vi "Add Elements to Meas Plugin UI.vi"(11 "error in (no error)":errorcluster) -> (15 "error out":errorcluster)   [LabVIEW 2021, in "Converter.lvlib"]
uses:
  Converter.lvlib
  Converter Reusables/Converter Reusables.lvlib
  Path Functions/Path Functions.lvlib
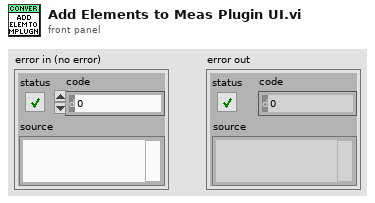
[diagram p1: front panel]
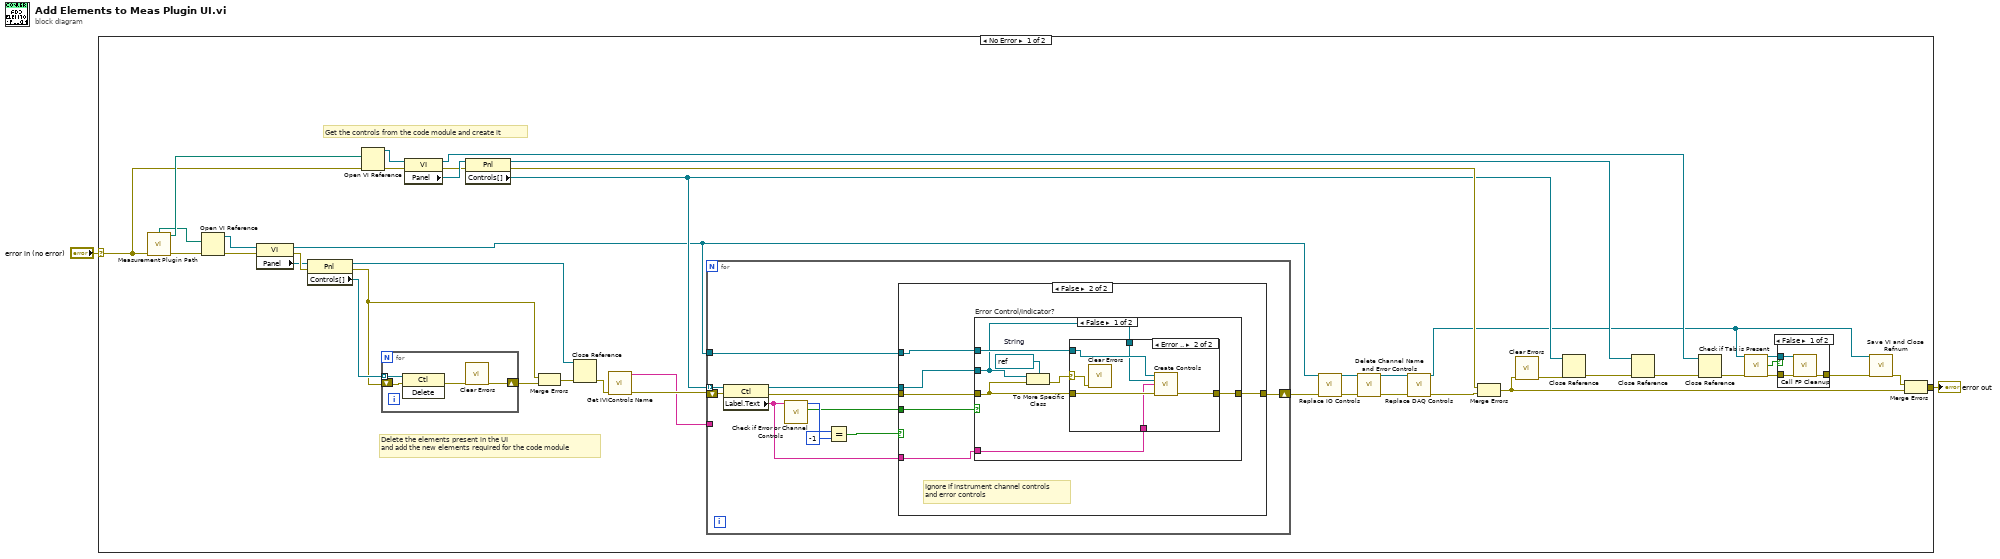
[diagram p0: block diagram]
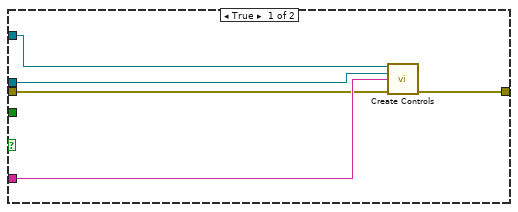
[diagram p2: hidden frame]
diagram:
  n1 = case shown="No Error" "error in (no error)" {
    selector: "error in (no error)" -> [w4 w91]
    tunnel: [w36 w91] -> w2
    frame No Error {
      # "Get the controls from the code module and create it"
      # "Delete the elements present in the UI\nand add the new elements required for the code module"
      n2 = call "Measurement Plugin Path.vi"("error in (no error)"=w4) -> ("Measurement UI"=w5:path, "New Code Module"=w6:path, "error out"=w3:errorcluster)  [unwired: 2 in, 10 out]
      n3 = Open VI Reference(vi path=w5, error in (no error)=w3) -> (vi reference=w24:refnum<vi>, error out=w45:errorcluster)  [unwired: 4 in]
      n4 = property class="VI"(reference=w24, error in=w45) -> (reference out=w28:refnum<vi>, error out=w44:errorcluster, "Panel"=w30:refnum<vi>)
      n5 = property class="Pnl"(reference=w30, error in=w44) -> (reference out=w29:refnum<vi>, error out=w15:errorcluster, "Controls[]"=w43:refnum<vi>[])
      n6 = Open VI Reference(vi path=w6, error in (no error)=w4) -> (vi reference=w21:refnum<vi>, error out=w38:errorcluster)  [unwired: 4 in]
      n7 = for {
        tunnel: w43 -> [w49] mode=indexing
        shift-right: [w46] -> w42
        shift-left: w15 -> [w48]
        n8 = invoke class="Ctl" method="Delete"(reference=w49, error in=w48) -> (error out=w47:errorcluster)  [unwired: 1 in, 2 out]
        n9 = call <vilib>:"Clear Errors.vi"("error in (no error)"=w47) -> ("error out"=w46:errorcluster)  [unwired: 5 in, 1 out]
      }
      n10 = property class="VI"(reference=w21, error in=w38) -> (reference out=w20:refnum<vi>, error out=w37:errorcluster, "Panel"=w39:refnum<vi>)
      n11 = property class="Pnl"(reference=w39, error in=w37) -> (reference out=w19:refnum<vi>, error out=w41:errorcluster, "Controls[]"=w40:refnum<vi>[])
      n12 = Merge Errors(w15, w42) -> (w16:errorcluster)
      n13 = Close Reference(reference=w29, error in (no error)=w16) -> (error out=w23:errorcluster)
      n14 = call "Get IVIControls Name.vi"("error in (no error)"=w23) -> ("Control Names Out"=w31:string[], "error out"=w32:errorcluster)  [unwired: 12 in, 1 out]
      n15 = for {
        tunnel: w28 -> [w60]
        tunnel: w40 -> [w58] mode=indexing
        shift-right: [w59] -> w27
        shift-left: w32 -> [w57]
        tunnel: w31 -> [_]
        n16 = property class="Ctl"(reference=w58, error in=w57) -> (reference out=w55:refnum<vi>, error out=w54:errorcluster, "Label.Text"=w56:string)
        n17 = call "Check if Error or Channel Controls.vi"("Label.Text"=w56) -> ("Error?"=w50:bool, "offset past match"=w53:i32)  [unwired: 9 in]
        n18 = Equal?(x=w53, y=-1) -> (x = y?=w51:bool)
        n19 = case shown="False" w51 {
          tunnel: w60 -> [w65 w68]
          tunnel: [w64 w66] -> w59
          tunnel: w55 -> [w62 w71]
          tunnel: w54 -> [w61 w70]
          tunnel: w56 -> [w63 w67]
          tunnel: w50 -> [_ w69]
          frame True {
            n20 = call "Create Controls.vi"("VI in"=w65, "Ctl Refnum"=w62, "Control Label"=w63, "error in (no error)"=w61) -> ("error out"=w64:errorcluster)  [unwired: 11 in]
          }
          frame False {
            # "Ignore if instrument channel controls\nand error controls"
            n21 = case "Error Control/Indicator?" shown="False" w69 {
              tunnel: w71 -> [w74 _]
              tunnel: w70 -> [w77 w86]
              tunnel: w68 -> [w75 _]
              tunnel: w67 -> [w73 _]
              tunnel: [w72 w86] -> w66
              frame False {
                w78 = refnum<vi> refnum  # String
                n22 = To More Specific Class(target class=w78, reference=w74, error in=w77) -> (error out=w76:errorcluster)  [unwired: 1 out]
                n23 = case shown="Error .." w76 {
                  selector: w76 -> [_ w80]
                  tunnel: w77 -> [w79 w85]
                  tunnel: w75 -> [_ w84]
                  tunnel: w74 -> [_ w83]
                  tunnel: w73 -> [_ w82]
                  tunnel: [w79 w81] -> w72
                  frame No Error {
                  }
                  frame Error {
                    n24 = call <vilib>:"Clear Errors.vi"("error in (no error)"=w80) -> ()  [unwired: 5 in, 2 out]
                    n25 = call "Create Controls.vi"("VI in"=w84, "Ctl Refnum"=w83, "Control Label"=w82, "error in (no error)"=w85) -> ("error out"=w81:errorcluster)  [unwired: 11 in]
                  }
                }
              }
              frame True {
              }
            }
          }
        }
      }
      n26 = call "Replace IO Controls.vi"("VI in"=w28, "error in (no error)"=w27) -> ("VI out"=w26:refnum<vi>, "error out"=w25:errorcluster)  [unwired: 12 in]
      n27 = call "Delete Channel Name and Error Controls.vi"("VI in"=w26, "error in (no error)"=w25) -> ("VI out"=w10:refnum<vi>, "error out"=w7:errorcluster)  [unwired: 12 in]
      n28 = call "Replace DAQ Controls.vi"("VI in"=w10, "error in (no error)"=w7) -> ("VI out"=w9:refnum<vi>, "error out"=w8:errorcluster)  [unwired: 12 in]
      n29 = Merge Errors(w41, w8) -> (w35:errorcluster)
      n30 = call <vilib>:"Clear Errors.vi"("error in (no error)"=w35) -> ("error out"=w34:errorcluster)  [unwired: 5 in, 1 out]
      n31 = Close Reference(reference=w40, error in (no error)=w34) -> (error out=w17:errorcluster)
      n32 = Close Reference(reference=w19, error in (no error)=w17) -> (error out=w18:errorcluster)
      n33 = Close Reference(reference=w20, error in (no error)=w18) -> (error out=w13:errorcluster)
      n34 = call "Check if Tab is Present.vi"("VI in"=w9, "error in (no error)"=w13) -> ("VI out"=w14:refnum<vi>, "Tab present?"=w11:bool, "error out"=w12:errorcluster)  [unwired: 11 in]
      n35 = case shown="False" w11 {
        tunnel: [w89 w90] -> w22
        tunnel: w14 -> [w88 _]
        tunnel: w12 -> [w87 w90]
        frame False {
          n36 = call "Call FP Cleanup.vi"("VI"=w88, "error in (no error)"=w87) -> ("error out"=w89:errorcluster)  [unwired: 13 in]
        }
        frame True {
        }
      }
      n37 = call "Save VI and Close Refnum.vi"("VI Refnum"=w9, "error in"=w22) -> ("error out"=w33:errorcluster)  [unwired: 13 in]
      n38 = Merge Errors(w33, w35) -> (w36:errorcluster)
    }
    frame Error {
    }
  }
  "error out" <- w2
